vi "Main Flush Current Action.vi"(8 "error in (no error)":errorcluster, 9 "Remaining Action":refnum<vi>, 10 "Action Finish Flg":refnum<vi>, 11 "error 2":refnum<vi>) -> (0 "error out":errorcluster)   [LabVIEW 2019]
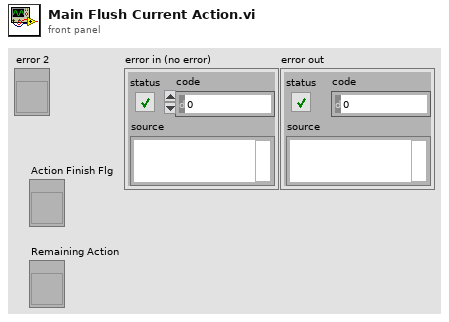
[diagram p1: front panel]
types:
  T1 = enum16{"Initial", "Add", "Read", "Delete & Check"}
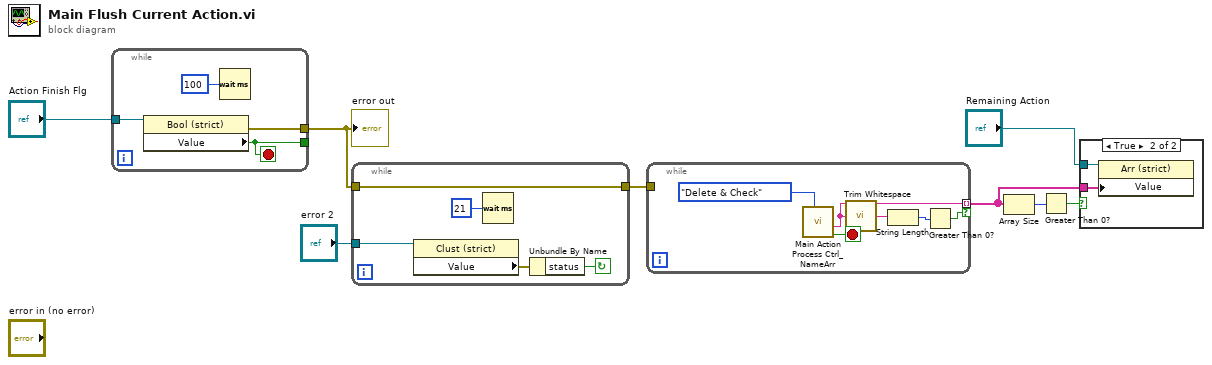
[diagram p0: block diagram]
diagram:
  n1 = while {
    tunnel: "Action Finish Flg" -> [w11]
    tunnel: [w10] -> _
    tunnel: [w9] -> w2
    stop <- w10 stop-if-true
    n2 = property on="Property Node" class="Bool (strict)"(reference=w11) -> (error out=w9:errorcluster, "Value"=w10:bool)  [unwired: 1 in, 1 out]
    n3 = Wait (ms)(milliseconds to wait=u32 100) -> ()  [unwired: 1 out]
  }
  "error out" <- w2
  n4 = while {
    tunnel: [w16] -> w3
    tunnel: w2 -> [w16]
    tunnel: "error 2" -> [w15]
    stop <- w13 continue-if-true
    n5 = property class="Clust (strict)"(reference=w15) -> ("Value"=w14:errorcluster)  [unwired: 1 in, 2 out]
    n6 = Wait (ms)(milliseconds to wait=u32 21) -> ()  [unwired: 1 out]
    n7 = Unbundle By Name(w14) -> ("status"=w13:bool)
  }
  n8 = while {
    tunnel: [w21] -> w7 mode=indexing if=w18
    tunnel: w3 -> [_]
    stop <- w22 stop-if-true
    n9 = call "Main Action Process Ctrl_NameArr.vi"("Action"=T1."Delete & Check") -> ("Finish"=w22:bool, "Delete Action"=w21:string)  [unwired: 6 in, 3 out]
    n10 = call <vilib>:"Trim Whitespace.vi"("string"=w21) -> ("trimmed string"=w20:string)  [unwired: 1 in]
    n11 = String Length(string=w20) -> (length=w19:i32)
    n12 = Greater Than 0?(x=w19) -> (x > 0?=w18:bool)
  }
  n13 = Array Size(array=w7) -> (size(s)=w6:i32)
  n14 = Greater Than 0?(x=w6) -> (x > 0?=w5:bool)
  n15 = case shown="True" w5 {
    tunnel: "Remaining Action" -> [_ w25]
    tunnel: w7 -> [_ w24]
    frame False {
    }
    frame True {
      n16 = property class="Arr (strict)"(reference=w25, "Value"=w24) -> ()  [unwired: 1 in, 2 out]
    }
  }
